vi "SSH_TUNNEL_ReadActivePorts.vi"(8 "error in (no error)":errorcluster, 11 "SSH_TUNNEL in":refnum<class "SSH_TUNNEL.lvclass">) -> (0 "error out":errorcluster, 1 "Local Ports forwarded to SSH":u16[](array[numeric]), 2 "MIDAS Destinations":u16[](array[numeric]), 3 "SSH_TUNNEL out":refnum<class "SSH_TUNNEL.lvclass">)   [LabVIEW 2018, in "feGEM DataPacker.lvlib" / "SSH_TUNNEL.lvclass"]
uses:
  SSH_TUNNEL.lvclass
  SSH_TUNNEL.lvclass/SSH_TUNNEL.ctl
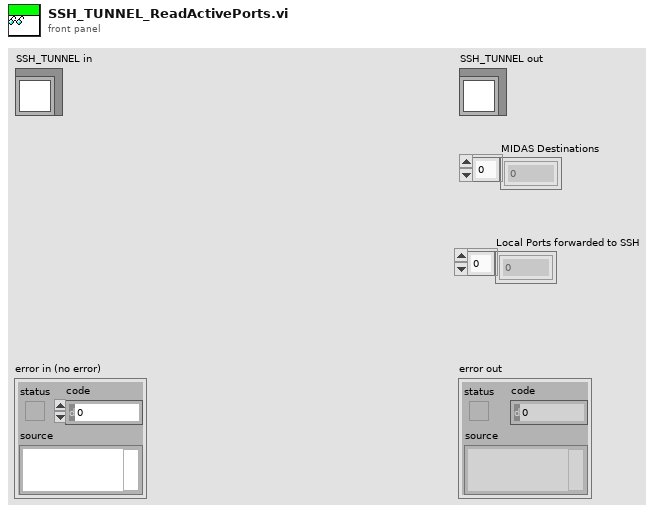
[diagram p1: front panel]
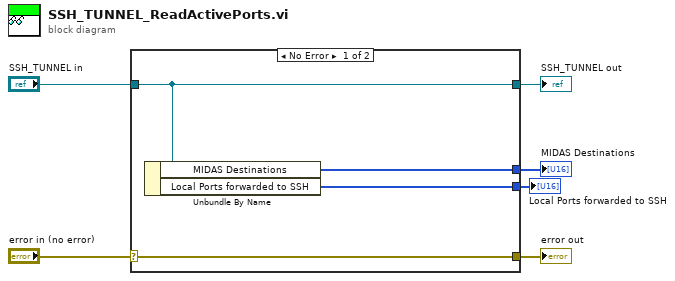
[diagram p0: block diagram]
diagram:
  n1 = case shown="No Error" "error in (no error)" {
    selector: "error in (no error)" -> [w10 w11]
    tunnel: [w10 w11] -> w5
    tunnel: [w9 w12] -> w3
    tunnel: "SSH_TUNNEL in" -> [w9 w12]
    tunnel: [w8 _] -> w2
    tunnel: [w7 _] -> w1
    frame No Error {
      n2 = Unbundle By Name(w9) -> ("MIDAS Destinations"=w8:u16[], "Local Ports forwarded to SSH"=w7:u16[])
    }
    frame Error {
    }
  }
  "error out" <- w5
  "SSH_TUNNEL out" <- w3
  "MIDAS Destinations" <- w2
  "Local Ports forwarded to SSH" <- w1
